vi "RG Get DAQ background level.vi"() -> ()   [LabVIEW 2014]
uses:
  <vilib>/Analysis/baseanly.llb/Mean (DBL).vi
  <vilib>/Analysis/NI_AALBase.lvlib
panel:
  out "Background level":dbl format="%0.5f"
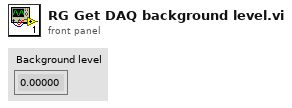
[diagram p1: front panel]
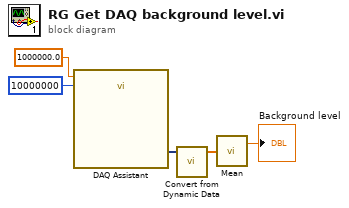
[diagram p0: block diagram]
diagram:
  n1 = call "DAQ Assistant"("rate"=1000000.0, "number of samples"=10000000) -> ("data"=w5:dynamicdata)  [unwired: 15 in, 2 out]
  n2 = call "Convert from Dynamic Data"("Dynamic Data Type"=w5) -> ("Array"=w4:dbl[])  [unwired: 3 in]
  n3 = call-poly <vilib>:"Mean.vi"("X"=w4) -> ("mean"=→"Background level":dbl)  [unwired: 1 out]
